vi "K2450 Ramp Jan2024.vi"() -> ()   [LabVIEW 2025]
doc: "Author: Scott Hannahs <sth@magnet.fsu.edu>\n\nThis software is licensed for use under the “MIT License\"\nCopyright (c) 2025 Scott Hannahs, sth@sth@magnet.sthnet.net\n\nPermission is hereby granted, free of charge, to any person obtaining a copy of this software and associated documentation files (the \"Software\"), to deal in the Software without restriction, including without limitation the rights to use, copy, modify, merge, publish, distribute, sublicense, and/or sell copies of the Software, and to permit persons to whom the Software is furnished to do so, subject to the following conditions: The above copyright notice and this permission notice shall be included in all copies or substantial portions of the Software.\n\nTHE SOFTWARE IS PROVIDED \"AS IS\", WITHOUT WARRANTY OF ANY KIND, EXPRESS OR IMPLIED, INCLUDING BUT NOT LIMITED TO THE WARRANTIES OF MERCHANTABILITY, FITNESS FOR A PARTICULAR PURPOSE AND NONINFRINGEMENT. IN NO EVENT SHALL THE AUTHORS OR COPYRIGHT HOLDERS BE LIABLE FOR ANY CLAIM, DAMAGES OR OTHER LIABILITY, WHETHER IN AN ACTION OF CONTRACT, TORT OR OTHERWISE, ARISING FROM, OUT OF OR IN CONNECTION WITH THE SOFTWARE OR THE USE OR OTHER DEALINGS IN THE SOFTWARE."
panel:
  in  "Mode":bool
  out "Time Remaining":dbl=60.0 format="%<%H:%M:%S>t"
  out "Output Value":dbl caption="Output Current" format="%_4g"
  in  "Time (Hr:Min:Sec)":dbl=60.0 step=1.0 format="%<%H:%M:%S>t"
  in  "Stop Value":dbl=0.01 caption="Stop Current" format="%_4g"
  in  "Start Ramp":bool
  in  "Cycle Time":dbl=0.1 format="%.3g"
  in  "stop":bool
  in  "VISA resource name":refnum<visa-resource-name>
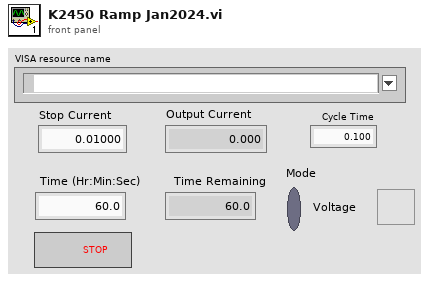
[diagram p1: front panel]
types:
  T1 = enum8{"Enabled", "Disabled", "Disabled and Grayed Out"}
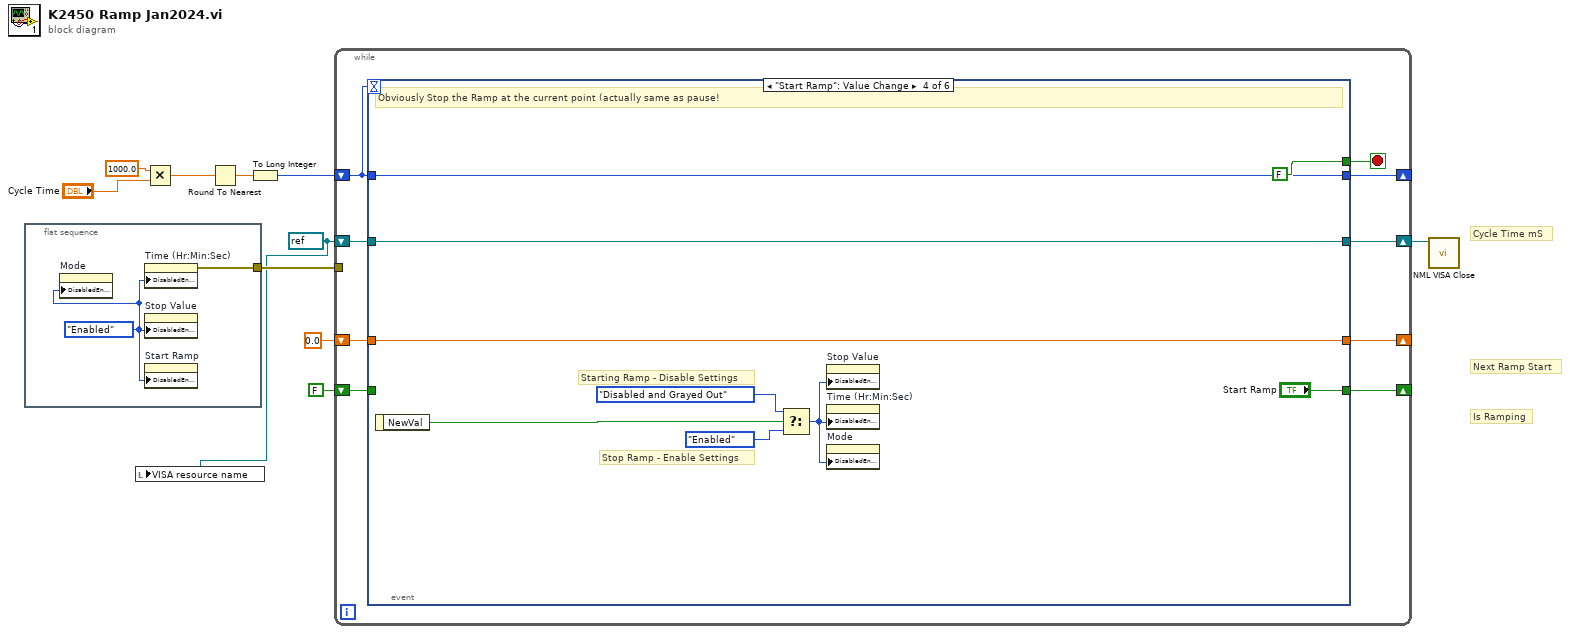
[diagram p0: block diagram]
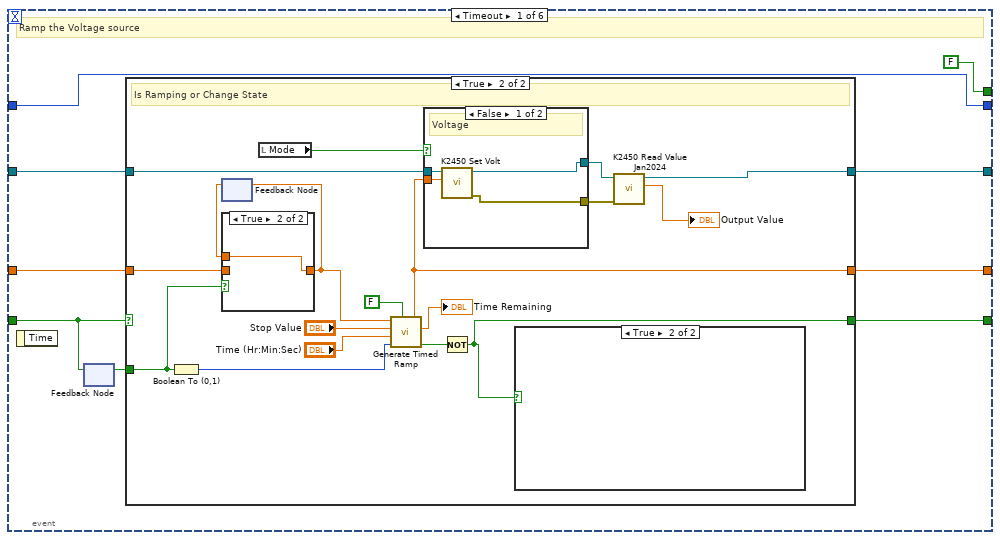
[diagram p2: hidden frame]
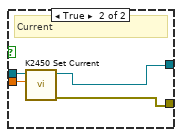
[diagram p4: hidden frame]
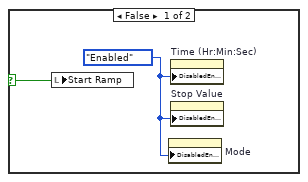
[diagram p6: hidden frame]
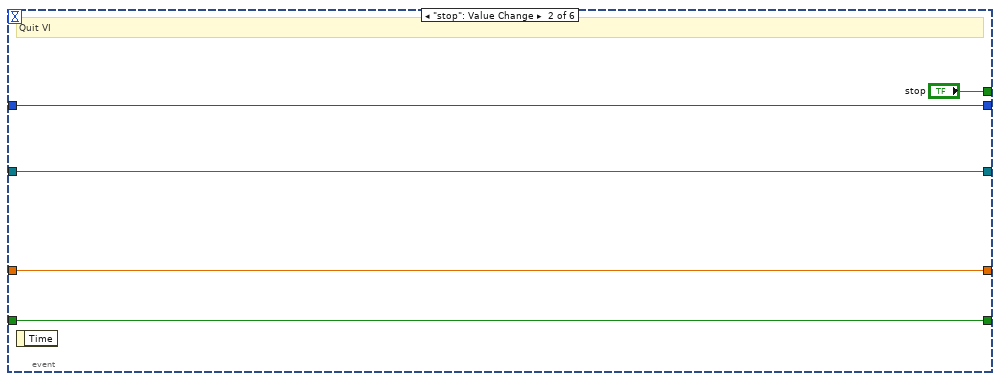
[diagram p7: hidden frame]
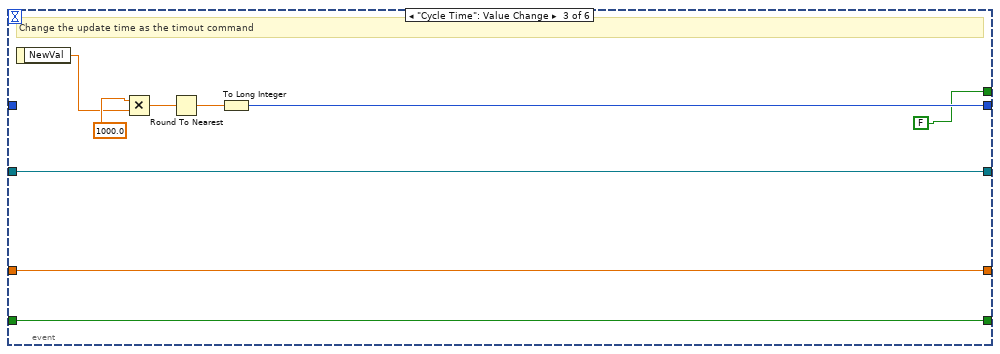
[diagram p8: hidden frame]
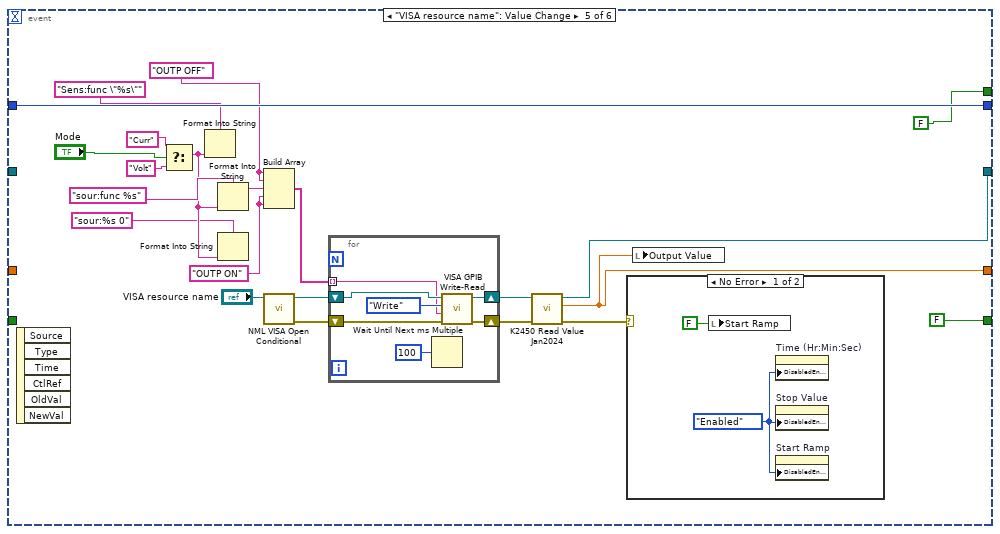
[diagram p9: hidden frame]
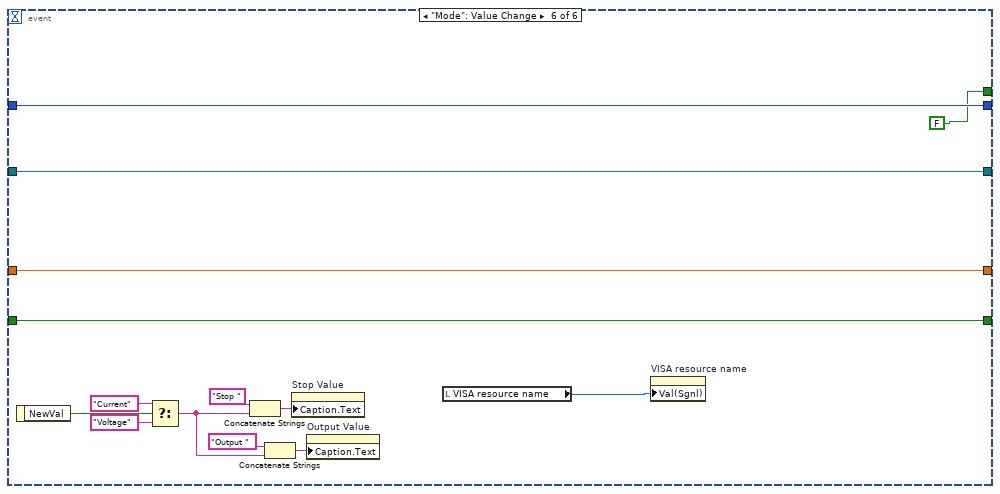
[diagram p11: hidden frame]
diagram:
  w1 = refnum<visa-resource-name> refnum ("dup VISA Session")
  # "Is Ramping"
  # "Next Ramp Start"
  # "Cycle Time mS"
  n1 = flat-sequence {
    tunnel: [w12] -> w2
    frame #0 {
      w11 = T1."Enabled" ("Disabled")
      n2 = property on="Mode" class="Bool (strict)"("DisabledEnum"=w11) -> ()  [unwired: 2 in, 2 out]
      n3 = property on="Time (Hr:Min:Sec)" class="DigNum (strict)"("DisabledEnum"=w11) -> (error out=w12:errorcluster)  [unwired: 2 in, 1 out]
      n4 = property on="Stop Value" class="DigNum (strict)"("DisabledEnum"=w11) -> ()  [unwired: 2 in, 2 out]
      n5 = property on="Start Ramp" class="Bool (strict)"("DisabledEnum"=w11) -> ()  [unwired: 2 in, 2 out]
    }
  }
  n6 = local write "VISA resource name"(w1) -> ()
  n7 = Multiply(x=1000.0, y="Cycle Time") -> (x*y=w9:dbl)
  n8 = Round To Nearest(number=w9) -> (nearest integer value=w7:dbl)
  n9 = To Long Integer(number=w7) -> (32bit integer=w6:i32)
  n10 = while {
    shift-right: [w17] -> w5
    shift-left: w1 -> [w18]
    shift-right: [w14] -> _
    shift-left: 0.0 ("Voitage 2450") -> [w13]
    shift-right: [w19] -> _
    shift-left: w6 -> [w20]
    shift-right: [w15] -> _
    shift-left: FALSE -> [w16]
    tunnel: w2 -> [_]
    stop <- w21 stop-if-true
    n11 = event shown="[3] \"Start Ramp\": Value Change" {
      selector: _ -> [_ _ _ _ _ _]
      dyn-events: _ -> [_ _ _ _ _ _]
      timeout: w20 -> [_ _ _ _ _ _]
      tunnel: [FALSE ("stop") "stop" FALSE ("stop") FALSE ("stop") FALSE ("stop") FALSE ("stop")] -> w21
      tunnel: w20 -> [w30 w67 _ w85 w102 w131]
      tunnel: [w30 w67 w73 w85 w102 w131] -> w19
      tunnel: w18 -> [w29 w64 w70 w84 _ w129]
      tunnel: [w28 w64 w70 w84 w103 w129] -> w17
      tunnel: w16 -> [w23 w66 w71 _ _ w127]
      tunnel: [w26 w66 w71 "Start Ramp" FALSE ("Start Ramp") w127] -> w15
      tunnel: [w24 w65 w69 w83 w99 w128] -> w14
      tunnel: w13 -> [w25 w65 w69 w83 _ w128]
      event Timeout {
        # "Ramp the Voltage source"
        n12 = event-data() -> ()  [unwired: 1 in, 1 out]
        n13 = feedback-in #1(w23) -> ()
        n14 = feedback #1() -> (w22:bool)  [unwired: 1 in]
        n15 = case shown="True" w23 {
          selector: w23 -> [w31 _]
          tunnel: w29 -> [w33 w50]
          tunnel: [w33 w34] -> w28
          tunnel: [w31 w44] -> w26
          tunnel: w25 -> [w32 w42]
          tunnel: [w32 w45] -> w24
          tunnel: w22 -> [_ w43]
          frame False {
            # "Idle"
          }
          frame True {
            # "Is Ramping or Change State"
            n16 = Boolean To (0,1)(Boolean=w43) -> (0, 1=w49:i16)
            n17 = feedback #2() -> (w40:dbl)  [unwired: 1 in]
            n18 = case shown="True" w43 {
              tunnel: w42 -> [w60 _]
              tunnel: [w60 w61] -> w41
              tunnel: w40 -> [_ w61]
              frame False {
              }
              frame True {
              }
            }
            n19 = feedback-in #2(w41) -> ()
            n20 = local read "Mode"() -> (w38:bool)
            n21 = call "Generate Timed Ramp.vi"("Log"=FALSE, "Point #"=w49, "Time (Hr:Min:Sec)"="Time (Hr:Min:Sec)", "Stop"="Stop Value", "Start"=w41) -> ("Stop"=w48:bool, "Time Remaining"=→"Time Remaining":dbl, "Output"=w45:dbl)  [unwired: 1 out]
            n22 = case shown="False" w38 {
              tunnel: w50 -> [w55 w59]
              tunnel: w45 -> [w54 w58]
              tunnel: [w53 w56] -> w37
              tunnel: [w52 w57] -> w36
              frame False {
                # "Voltage"
                n23 = call "K2450 Set Volt.vi"("Voltage 2450"=w54, "VISA resource name"=w55) -> ("error out"=w53:errorcluster, "dup VISA Session"=w52:refnum<visa-resource-name>)  [unwired: 7 in, 1 out]
              }
              frame True {
                # "Current"
                n24 = call "K2450 Set Current.vi"("Current 2450"=w58, "VISA resource name"=w59) -> ("error out"=w56:errorcluster, "dup VISA Session"=w57:refnum<visa-resource-name>)  [unwired: 8 in]
              }
            }
            n25 = Not(x=w48) -> (.not. x?=w44:bool)
            n26 = case shown="True" w44 {
              selector: w44 -> [w63 _]
              frame False {
                w62 = T1."Enabled" ("Disabled")
                n27 = local write "Start Ramp"(w63) -> ()
                n28 = property on="Mode" class="Bool (strict)"("DisabledEnum"=w62) -> ()  [unwired: 2 in, 2 out]
                n29 = property on="Time (Hr:Min:Sec)" class="DigNum (strict)"("DisabledEnum"=w62) -> ()  [unwired: 2 in, 2 out]
                n30 = property on="Stop Value" class="DigNum (strict)"("DisabledEnum"=w62) -> ()  [unwired: 2 in, 2 out]
              }
              frame True {
              }
            }
            n31 = call "K2450 Read Value Jan2024.vi"("error in (no error)"=w37, "VISA resource name"=w36) -> ("Value 2450"=→"Output Value":dbl, "dup VISA Session"=w34:refnum<visa-resource-name>)  [unwired: 7 in, 1 out]
          }
        }
      }
      event "stop": Value Change {
        # "Quit VI"
        n32 = event-data() -> ()  [unwired: 1 in, 1 out]
      }
      event "Cycle Time": Value Change {
        # "Change the update time as the timout command"
        n33 = event-data() -> ("NewVal"=w74:dbl)  [unwired: 1 in]
        n34 = Multiply(x=1000.0, y=w74) -> (x*y=w75:dbl)
        n35 = Round To Nearest(number=w75) -> (nearest integer value=w77:dbl)
        n36 = To Long Integer(number=w77) -> (32bit integer=w73:i32)
      }
      event "Start Ramp": Value Change {
        # "Stop Ramp - Enable Settings"
        # "Starting Ramp - Disable Settings"
        # "Obviously Stop the Ramp at the current point (actually same as pause!"
        n37 = event-data() -> ("NewVal"=w81:bool)  [unwired: 1 in]
        n38 = Select(t=T1."Disabled and Grayed Out" ("Disabled"), s=w81, f=T1."Enabled" ("Disabled")) -> (s? t:f=w78:T1)
        n39 = property on="Stop Value" class="DigNum (strict)"("DisabledEnum"=w78) -> ()  [unwired: 2 in, 2 out]
        n40 = property on="Time (Hr:Min:Sec)" class="DigNum (strict)"("DisabledEnum"=w78) -> ()  [unwired: 2 in, 2 out]
        n41 = property on="Mode" class="Bool (strict)"("DisabledEnum"=w78) -> ()  [unwired: 2 in, 2 out]
      }
      event "VISA resource name": Value Change {
        w88 = "OUTP OFF"
        w87 = "OUTP ON"
        n42 = event-data() -> ()  [unwired: 1 in, 6 out]
        n43 = Select(t="Curr", s="Mode", f="Volt") -> (s? t:f=w92:string)
        n44 = Format Into String(format string="Sens:func \"%s\"", w92) -> ()  [unwired: 2 in, 2 out]
        n45 = Format Into String(format string="sour:func %s", w92) -> (resulting string=w93:string)  [unwired: 2 in, 1 out]
        n46 = Format Into String(format string="sour:%s 0" ("initial string"), w92) -> ()  [unwired: 2 in, 2 out]
        n47 = Build Array(w88, w88, w93, w87, w87) -> (w90:string[])
        n48 = call "NML VISA Open Conditional.vi"("VISA resource name"="VISA resource name") -> ("error out"=w108:errorcluster, "dup VISA Session"=w105:refnum<visa-resource-name>)  [unwired: 8 in, 1 out]
        n49 = for {
          shift-right: [w115] -> w106
          shift-left: w105 -> [w113]
          shift-right: [w116] -> w107
          shift-left: w108 -> [w114]
          tunnel: w90 -> [w112] mode=indexing
          n50 = Wait Until Next ms Multiple(millisecond multiple=u32 100) -> ()  [unwired: 1 out]
          n51 = call "VISA GPIB Write-Read.vi"("error in (no error)"=w114, "Command"=w112, "Action"=enum16{"Write", "Read", "Write & Read"}."Write", "VISA resource name"=w113) -> ("error out"=w116:errorcluster, "dup VISA Session"=w115:refnum<visa-resource-name>)  [unwired: 4 in, 2 out]
        }
        n52 = call "K2450 Read Value Jan2024.vi"("error in (no error)"=w107, "VISA resource name"=w106) -> ("error out"=w100:errorcluster, "Value 2450"=w99:dbl, "dup VISA Session"=w103:refnum<visa-resource-name>)  [unwired: 7 in]
        n53 = case shown="No Error" w100 {
          frame No Error {
            w110 = T1."Enabled" ("Disabled")
            n54 = local write "Start Ramp"(FALSE ("Start Ramp")) -> ()
            n55 = property on="Time (Hr:Min:Sec)" class="DigNum (strict)"("DisabledEnum"=w110) -> ()  [unwired: 2 in, 2 out]
            n56 = property on="Stop Value" class="DigNum (strict)"("DisabledEnum"=w110) -> ()  [unwired: 2 in, 2 out]
            n57 = property on="Start Ramp" class="Bool (strict)"("DisabledEnum"=w110) -> ()  [unwired: 2 in, 2 out]
          }
          frame Error {
          }
        }
        n58 = local write "Output Value"(w99) -> ()
      }
      event "Mode": Value Change {
        n59 = event-data() -> ("NewVal"=w121:bool)  [unwired: 1 in]
        n60 = Select(t="Current" ("string"), s=w121, f="Voltage" ("string")) -> (s? t:f=w122:string)
        n61 = Concatenate Strings("Stop " ("string"), w122) -> (w124:string)
        n62 = Concatenate Strings("Output " ("string"), w122) -> (w123:string)
        n63 = property on="Stop Value" class="DigNum (strict)"("Caption.Text"=w124) -> ()  [unwired: 2 in, 2 out]
        n64 = property on="Output Value" class="DigNum (strict)"("Caption.Text"=w123) -> ()  [unwired: 2 in, 2 out]
        n65 = local read "VISA resource name"() -> (w118:refnum<visa-resource-name>)
        n66 = property on="VISA resource name" class="VISAName"("Val(Sgnl)"=w118) -> ()  [unwired: 2 in, 2 out]
      }
    }
  }
  n67 = call "NML VISA Close.vi"("VISA resource name"=w5) -> ()  [unwired: 10 in, 1 out]
